vi "PupilTracker.vi"() -> ()   [LabVIEW 2013]
uses:
  PupilTrackerStates.ctl
  <vilib>/vision/NI_Vision_Development_Module.lvlib
  <vilib>/vision/Image Controls.llb/IMAQ Image.ctl
panel:
  in  "Tab Control":T1(tab)
  out "Pupil marked":bool=TRUE
  out "Saving Pupil Video":bool=TRUE
  out "LostFrames":u32
  out "Tracking Pupil":bool
  out "PupilCamera":T2(plugin-control)
  out "Frame Rate Eyetracker":dbl
  out "Avg freq":dbl caption="Eyetracker - Mean \nprocessing frequency (Hz)" format="%0.2f"
  out "Pupil Info":T3(graph)
  in  "Storage Folder":path
  in  "Save Block Video":bool
  in  "Track Pupil":bool
  in  "Rescan Image":bool=TRUE
  in  "Select Pupil Area":bool
  in  "Pupil Camera":bool=TRUE
  in  "Acquisition Frame Rate":dbl=30.0 min=1.0 max=100000.0
  out "Processed":T2(plugin-control)
  in  "Manual Threshold":cluster{sgl, sgl}(slide)={0.0, 150.0} caption="Threshold Range" scale=0.0..255.0
  in  "Track Every Nth Frame":i32=1
  in  "Exposure Time":dbl(slide)=7611.0 min=10.0 max=850000.0 scale=1000.0..10000.0
  in  "Gain":dbl(slide)=7.281634828221404 min=0.0 max=24.014274679280266 scale=0.0..10.0
  in  "Black Level":dbl(slide)=-17.75 min=-32.0 max=31.75 scale=-30.0..30.0
  in  "BtnQuit":bool
  out "Processed Image Display":T2
  out "Stop Acquisition":bool=TRUE
  out "Vision Acquisition Error":errorcluster
  out "Paused Acquisition":bool=TRUE
  out "Fitted Pupil Image":T2
  out "Last Image number":u32
  in  "Save Tracking Results":bool=TRUE
  out "Pupil Frame No":i32
  out "Processed Image":T2
  out "Cropped Image":T2
  out "Exit program":bool
  # "Camera Connection"
  # "Start Tracking"
  # "Optimize Tracking"
  # "Tracker Settings"
  # "Set tracker to rescan entire image if pupil is not found within search area"
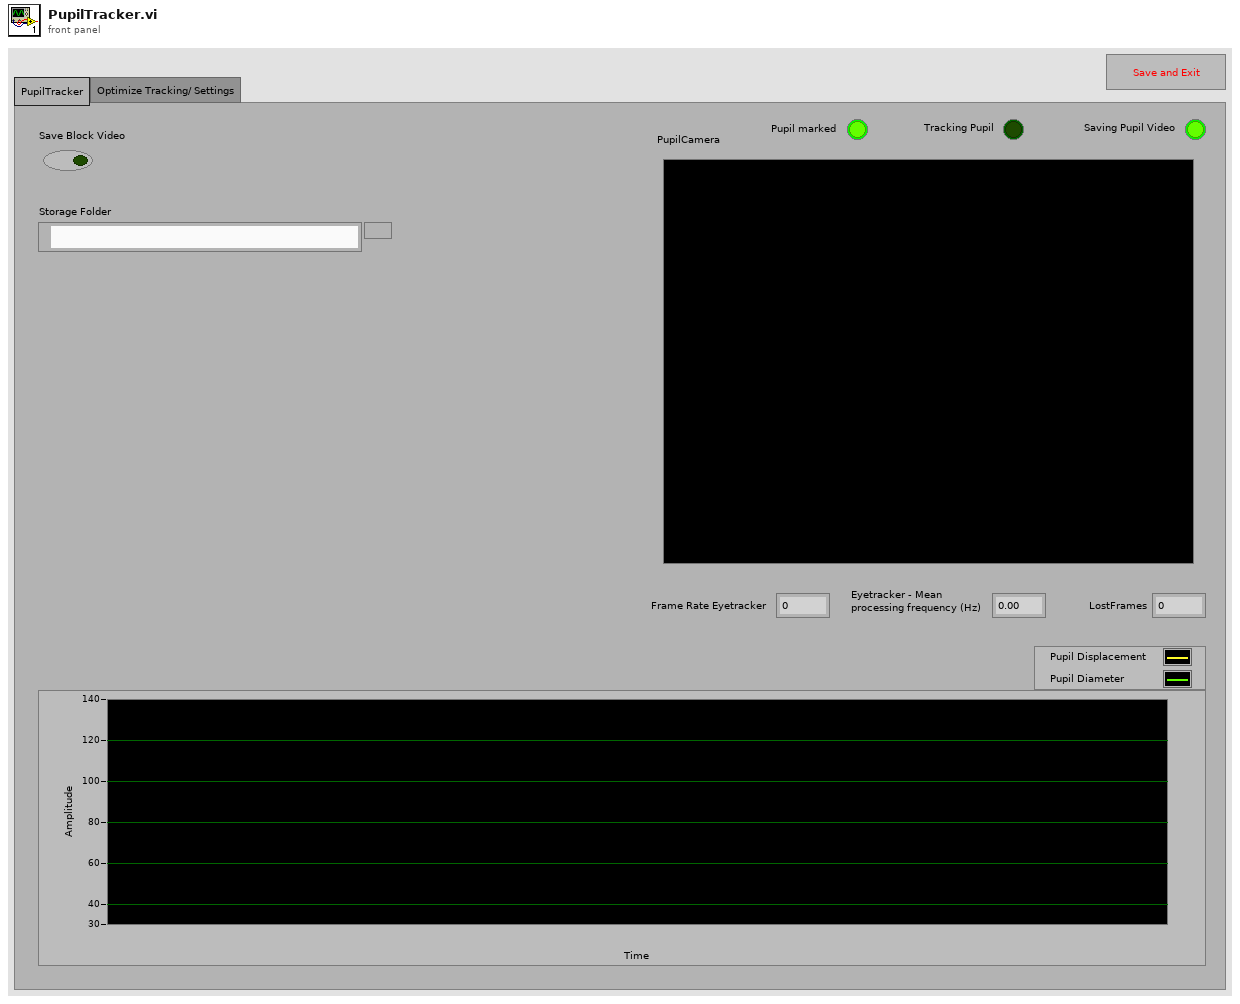
[diagram p1: front panel]
types:
  T1 = enum32{"PupilTracker", "Optimize Tracking/ Settings"}
  T2 = typedef "IMAQ Image.ctl" = refnum<image>
  T3 = cluster{"Numeric":dbl, "Average of last N array elements":dbl}
  T4 = typedef "PupilTrackerStates.ctl" = enum16{"Initialize Eyetracker", "Idle", "Run Acquisition", "Update Acquisition Parameters", "Camera Error", "Pupil Unmarked Error", "Quit Eyetracker"}
  T5 = cluster{"Numeric":dbl, "Average of last N array elements":dbl}[]
  T6 = typedef "Image Type" = u32
  T7 = cluster{"Frame No":i32, "Circle time series":dbl[][], "Rectangle coordinates":i32[], "Annulus ROI":cluster{"ID":enum32{"External", "Internal"}, "Type":u32, i32[]}, "Annulus coordinates":i32[]}
  T8 = cluster{"Pupil Displacement":dbl, "Average Pupil Diameter":dbl}
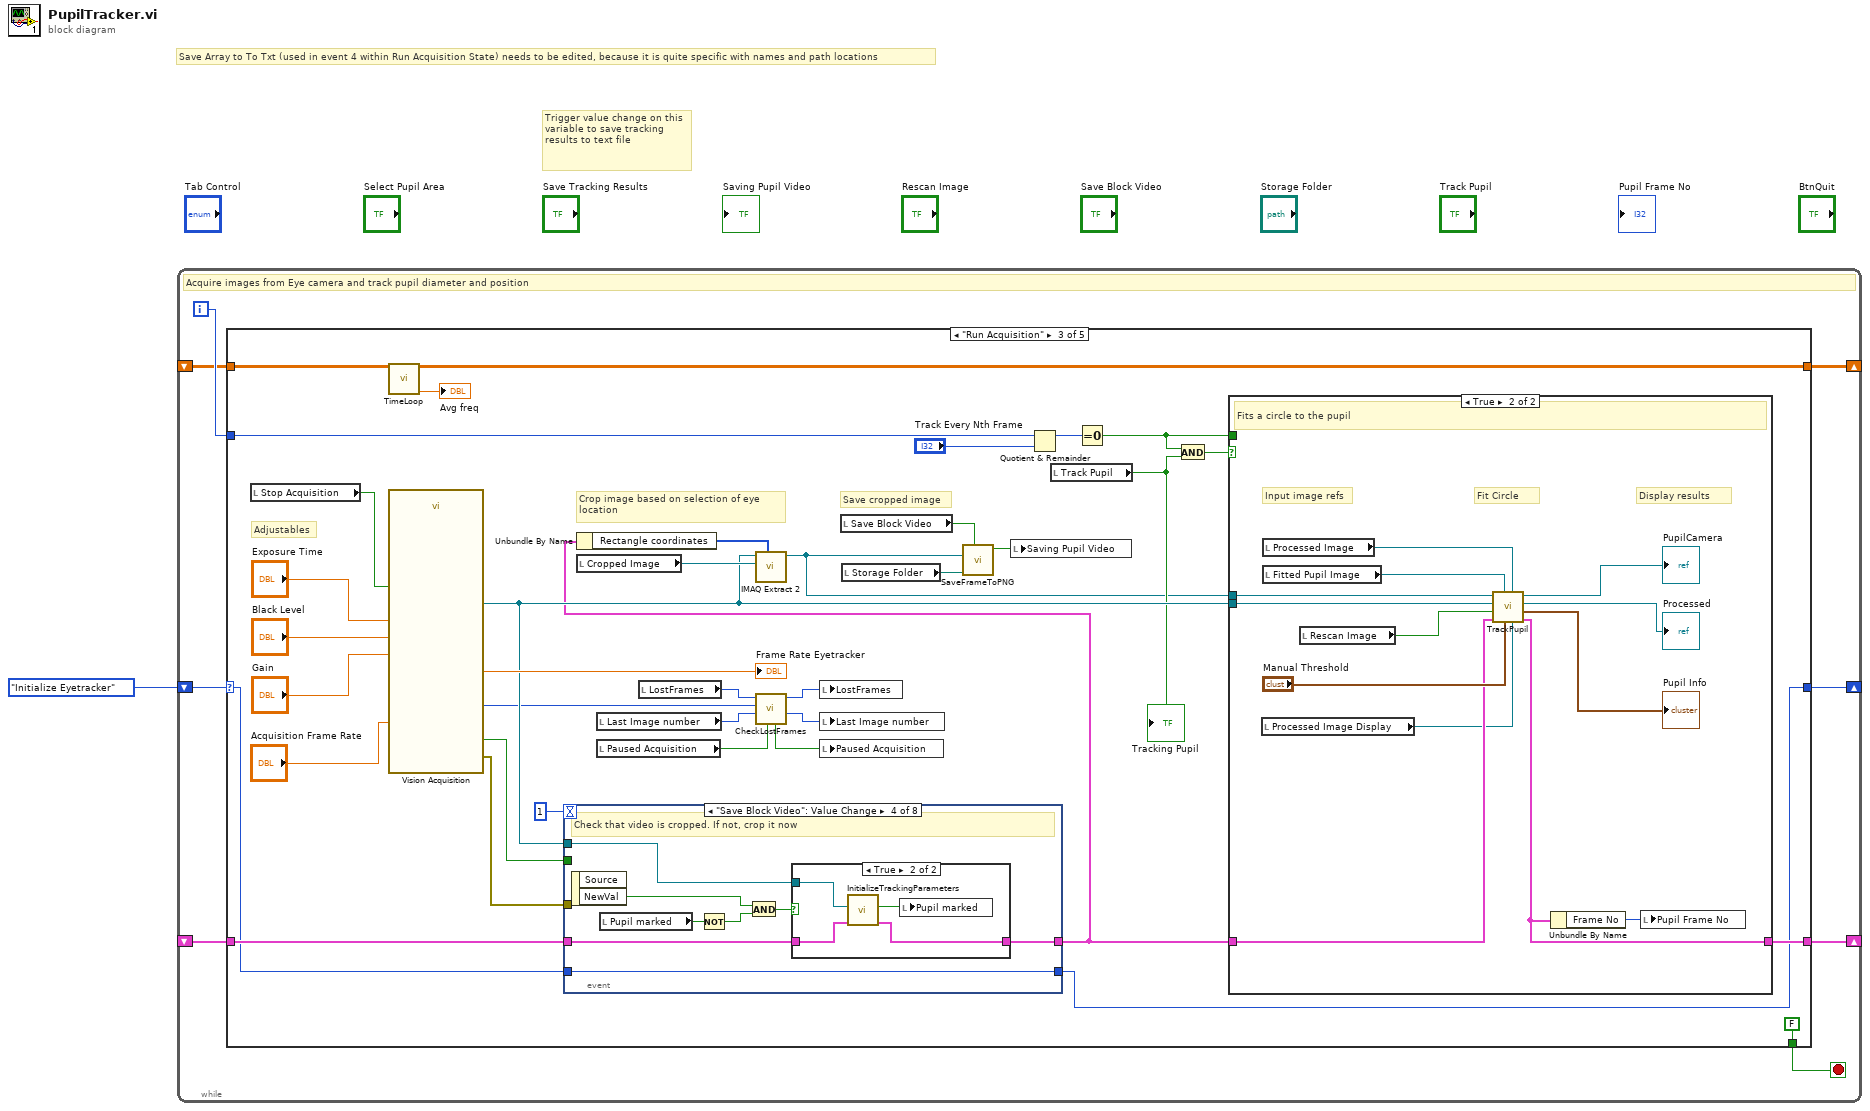
[diagram p0: block diagram]
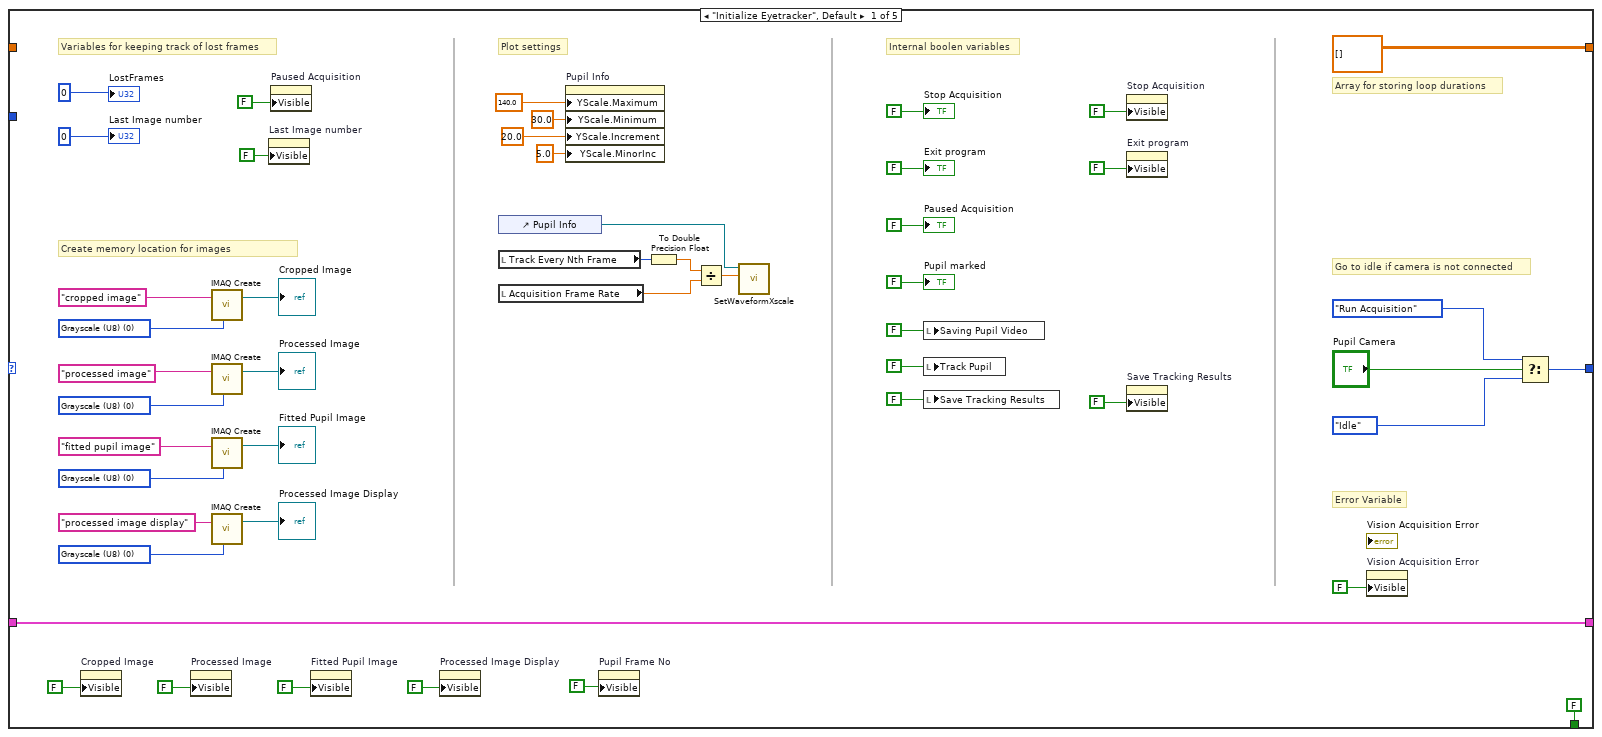
[diagram p2: hidden frame]
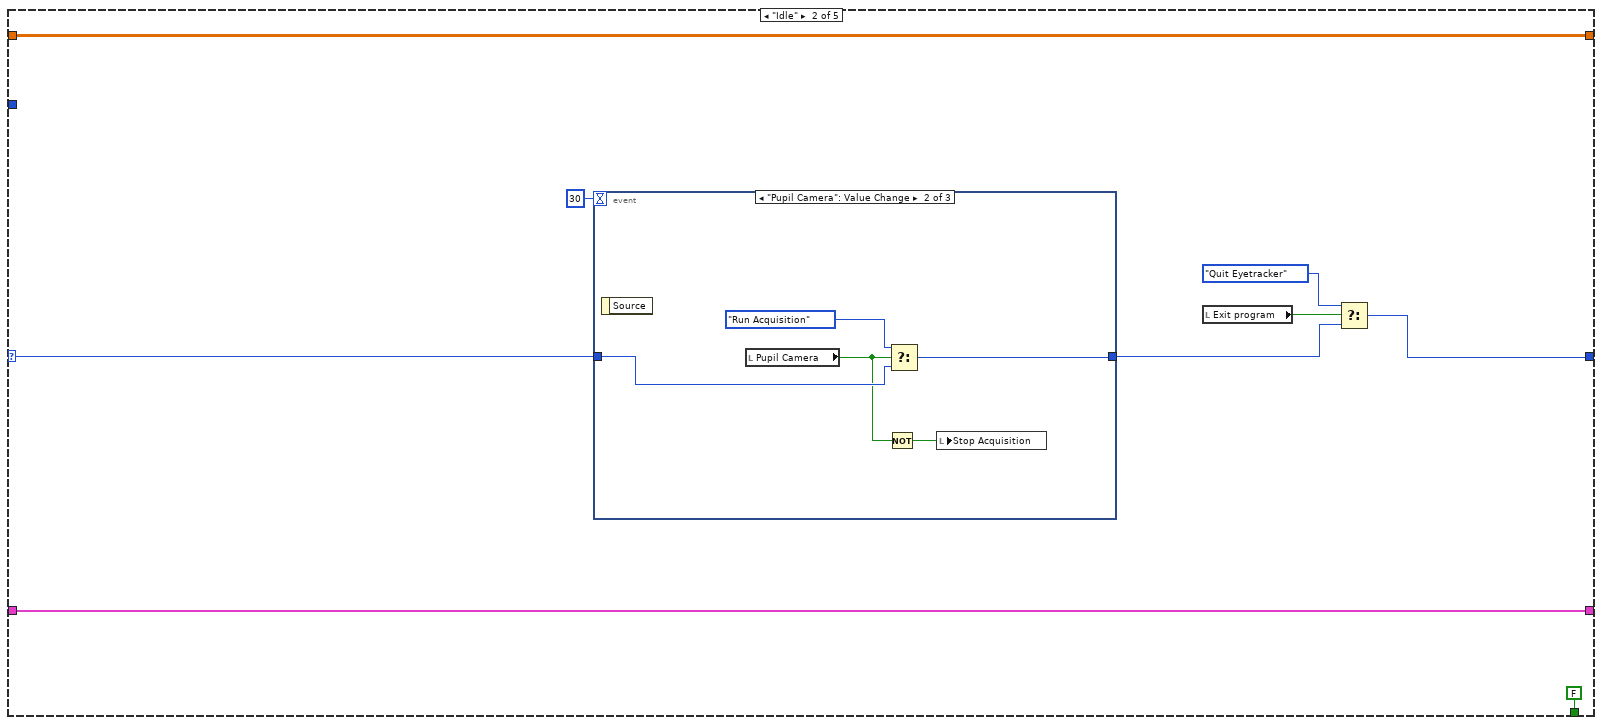
[diagram p3: hidden frame]
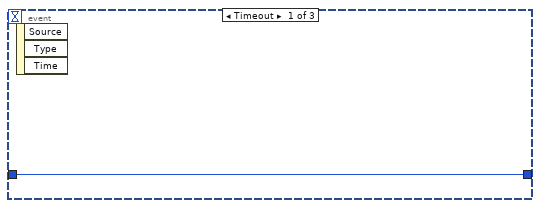
[diagram p4: hidden frame]
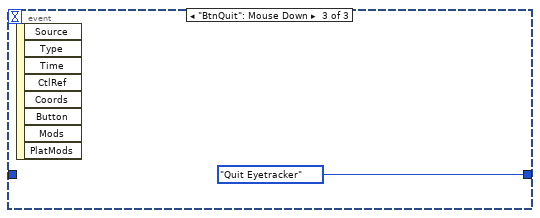
[diagram p5: hidden frame]
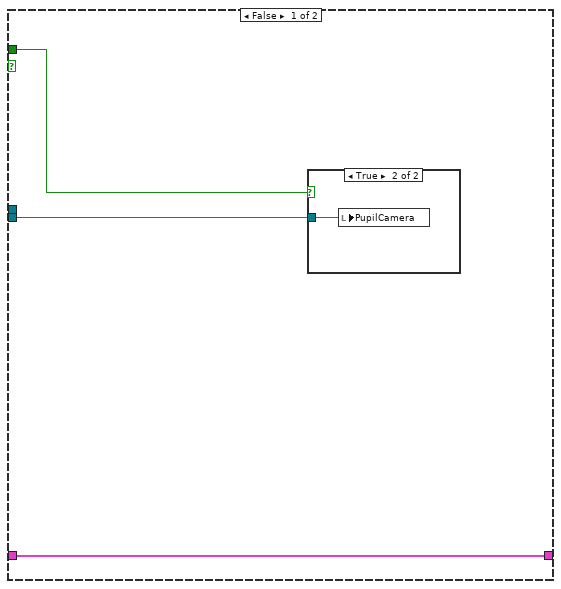
[diagram p6: hidden frame]
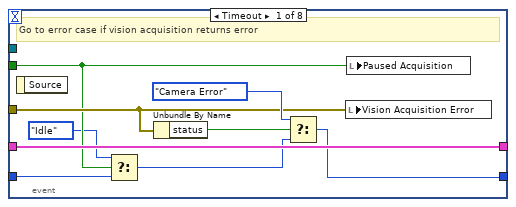
[diagram p8: hidden frame]
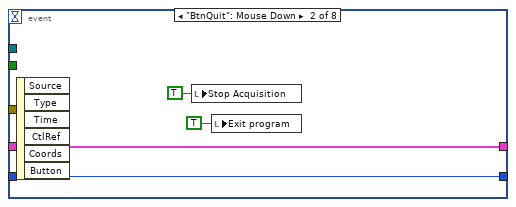
[diagram p9: hidden frame]
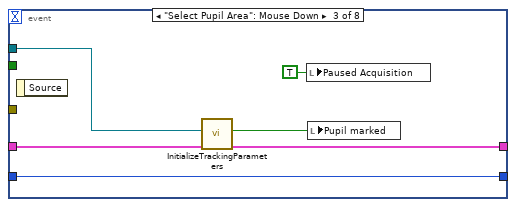
[diagram p10: hidden frame]
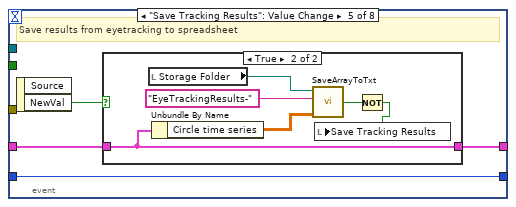
[diagram p12: hidden frame]
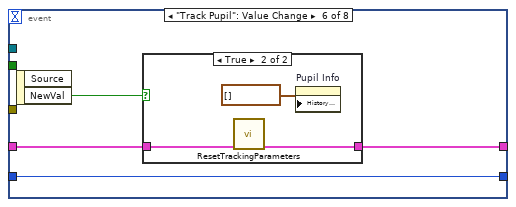
[diagram p14: hidden frame]
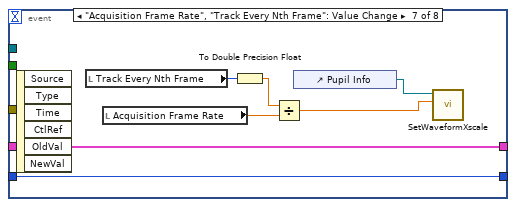
[diagram p16: hidden frame]
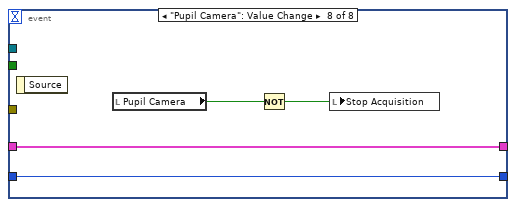
[diagram p17: hidden frame]
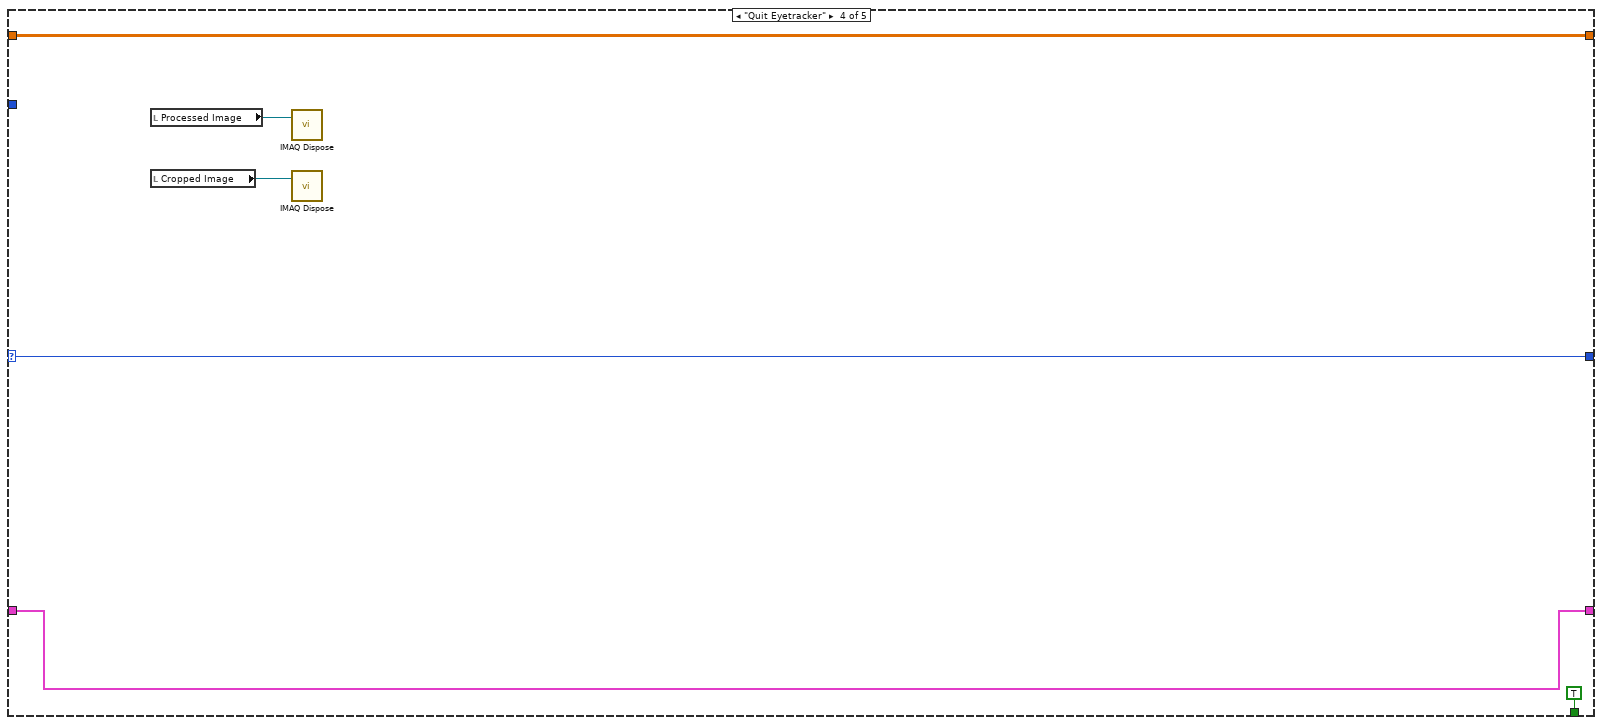
[diagram p18: hidden frame]
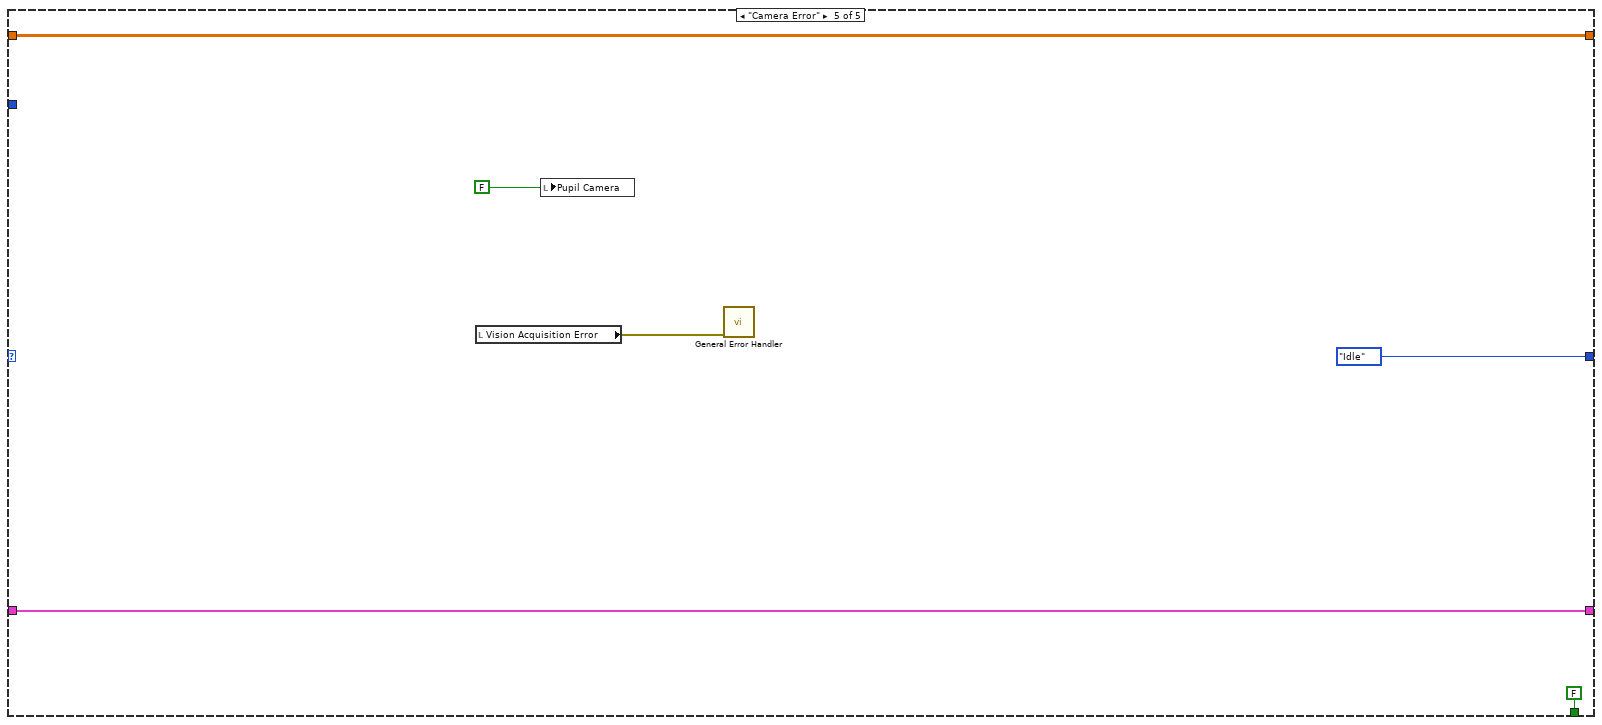
[diagram p19: hidden frame]
diagram:
  # "Save Array to To Txt (used in event 4 within Run Acquisition State) needs to be edited, because it is quite specific with names and path locations"
  # "Trigger value change on this variable to save tracking results to text file"
  n1 = while {
    shift-right: [w5] -> _
    shift-left: _ -> [w6]
    shift-right: [w9] -> _
    shift-left: _ -> [w7]
    shift-right: [w2] -> _
    shift-left: PupilTrackerStates."Initialize Eyetracker" -> [w3]
    i -> [w8]
    stop <- w4 stop-if-true
    # "Acquire images from Eye camera and track pupil diameter and position"
    n2 = case shown="\"Run Acquisition\"" w3 {
      selector: w3 -> [_ w62 w84 w193 _]
      tunnel: [w57 w65 w110 w191 w200] -> w9
      tunnel: w8 -> [_ _ w109 _ _]
      tunnel: w7 -> [w57 w65 w104 w191 w200]
      tunnel: w6 -> [_ w66 w92 w196 w201]
      tunnel: [dbl[][] [] w66 w91 w196 w201] -> w5
      tunnel: [w55 w59 w83 w193 PupilTrackerStates."Idle"] -> w2
      tunnel: [FALSE ("Stopped") FALSE ("Stopped") FALSE ("Stopped") TRUE ("Stopped") FALSE ("Stopped")] -> w4
      frame "Initialize Eyetracker", Default {
        w29 = T6 0 items=["Grayscale (U8)", "Grayscale (I16)", "Grayscale (SGL)", "Complex (CSG)", "RGB (U32)", "HSL (U32)", "RGB (U64)", "Grayscale (U16)"] ("Image Type")
        w48 = T6 0 items=["Grayscale (U8)", "Grayscale (I16)", "Grayscale (SGL)", "Complex (CSG)", "RGB (U32)", "HSL (U32)", "RGB (U64)", "Grayscale (U16)"] ("Image Type")
        w51 = T6 0 items=["Grayscale (U8)", "Grayscale (I16)", "Grayscale (SGL)", "Complex (CSG)", "RGB (U32)", "HSL (U32)", "RGB (U64)", "Grayscale (U16)"] ("Image Type")
        w53 = T6 0 items=["Grayscale (U8)", "Grayscale (I16)", "Grayscale (SGL)", "Complex (CSG)", "RGB (U32)", "HSL (U32)", "RGB (U64)", "Grayscale (U16)"] ("Image Type")
        # "Error Variable"
        # "Internal boolen variables"
        # "Plot settings"
        # "Go to idle if camera is not connected"
        # "Variables for keeping track of lost frames"
        # "Create memory location for images"
        # "Array for storing loop durations"
        n3 = property on="Cropped Image" class="IMAQImage (strict)"("Visible"=FALSE) -> ()  [unwired: 2 in, 2 out]
        n4 = property on="Processed Image" class="IMAQImage (strict)"("Visible"=FALSE) -> ()  [unwired: 2 in, 2 out]
        n5 = call "IMAQ Create"("Image Name"="cropped image", "Image Type"=w53) -> ("New Image"=→"Cropped Image":T2)  [unwired: 3 in, 1 out]
        n6 = call "IMAQ Create"("Image Name"="processed image", "Image Type"=w51) -> ("New Image"=→"Processed Image":T2)  [unwired: 3 in, 1 out]
        n7 = call "IMAQ Create"("Image Name"="fitted pupil image", "Image Type"=w48) -> ("New Image"=→"Fitted Pupil Image":T2)  [unwired: 3 in, 1 out]
        n8 = call "IMAQ Create"("Image Name"="processed image display", "Image Type"=w29) -> ("New Image"=→"Processed Image Display":T2)  [unwired: 3 in, 1 out]
        n9 = property on="Last Image number" class="DigNum (strict)"("Visible"=FALSE) -> ()  [unwired: 2 in, 2 out]
        n10 = property on="Paused Acquisition" class="Bool (strict)"("Visible"=FALSE) -> ()  [unwired: 2 in, 2 out]
        n11 = property on="Fitted Pupil Image" class="IMAQImage (strict)"("Visible"=FALSE) -> ()  [unwired: 2 in, 2 out]
        n12 = property on="Processed Image Display" class="IMAQImage (strict)"("Visible"=FALSE) -> ()  [unwired: 2 in, 2 out]
        n13 = control-ref of="Pupil Info"() -> (w30:refnum<vi>)
        n14 = local read "Track Every Nth Frame"() -> (w40:i32)
        n15 = local read "Acquisition Frame Rate"() -> (w41:dbl)
        n16 = property on="Pupil Info" class="WFChart (strict)"("YScale.Maximum"=140.0 ("Y Scale.Range:Increment"), "YScale.Minimum"=30.0 ("Y Scale.Range:Maximum"), "YScale.Increment"=20.0 ("Y Scale.Range:Minimum"), "YScale.MinorInc"=5.0 ("Y Scale.Range:Minor Increment")) -> ()  [unwired: 2 in, 2 out]
        n17 = property on="Pupil Frame No" class="DigNum (strict)"("Visible"=FALSE) -> ()  [unwired: 2 in, 2 out]
        n18 = To Double Precision Float(number=w40) -> (double precision float=w39:dbl)
        n19 = Divide(x=w39, y=w41) -> (x/y=w33:dbl)
        n20 = call "SetWaveformXscale.vi"("deltaT"=w33, "WaveformChart in"=w30) -> ()  [unwired: 10 in]
        n21 = local write "Saving Pupil Video"(FALSE ("Saving Pupil Video")) -> ()
        n22 = local write "Track Pupil"(FALSE ("Track Pupil")) -> ()
        n23 = local write "Save Tracking Results"(FALSE ("Save Tracking Results")) -> ()
        n24 = property on="Stop Acquisition" class="Bool (strict)"("Visible"=FALSE) -> ()  [unwired: 2 in, 2 out]
        n25 = property on="Exit program" class="Bool (strict)"("Visible"=FALSE) -> ()  [unwired: 2 in, 2 out]
        n26 = property on="Save Tracking Results" class="Bool (strict)"("Visible"=FALSE) -> ()  [unwired: 2 in, 2 out]
        n27 = property on="Vision Acquisition Error" class="Clust (strict)"("Visible"=FALSE) -> ()  [unwired: 2 in, 2 out]
        n28 = Select(t=PupilTrackerStates."Run Acquisition", s="Pupil Camera", f=PupilTrackerStates."Idle") -> (s? t:f=w55:T4)
        "Last Image number" <- u32 0 ("Last Image number")
        "LostFrames" <- u32 0 ("LostFrames")
        "Paused Acquisition" <- FALSE ("Paused Acquisition")
        "Exit program" <- FALSE ("Exit program")
        "Stop Acquisition" <- FALSE ("Stop Acquisition")
        "Pupil marked" <- FALSE ("Pupil marked")
      }
      frame "Idle" {
        n29 = event shown="[1] \"Pupil Camera\": Value Change" {
          selector: _ -> [_ _ _]
          dyn-events: _ -> [_ _ _]
          timeout: 30 -> [_ _ _]
          tunnel: [w67 w72 PupilTrackerStates."Quit Eyetracker"] -> w60
          tunnel: w62 -> [w67 w71 _]
          event Timeout {
            n30 = event-data() -> ()  [unwired: 1 in, 3 out]
          }
          event "Pupil Camera": Value Change {
            n31 = event-data() -> ()  [unwired: 1 in, 1 out]
            n32 = local read "Pupil Camera"() -> (w68:bool)
            n33 = Not(x=w68) -> (.not. x?=w69:bool)
            n34 = Select(t=PupilTrackerStates."Run Acquisition", s=w68, f=w71) -> (s? t:f=w72:T4)
            n35 = local write "Stop Acquisition"(w69) -> ()
          }
          event "BtnQuit": Mouse Down {
            n36 = event-data() -> ()  [unwired: 1 in, 8 out]
          }
        }
        n37 = local read "Exit program"() -> (w61:bool)
        n38 = Select(t=PupilTrackerStates."Quit Eyetracker", s=w61, f=w60) -> (s? t:f=w59:T4)
      }
      frame "Run Acquisition" {
        # "Save cropped image"
        # "Crop image based on selection of eye location"
        # "Adjustables"
        n39 = local read "Stop Acquisition"() -> (w79:bool)
        n40 = call "TimeLoop.vi"("Loop durations in"=w92) -> ("Average fps"=→"Avg freq":dbl, "Loop durations out"=w91:dbl[][])  [unwired: 5 in]
        n41 = call "Vision Acquisition"("Analog Control::Gain"="Gain", "Analog Control::Black Level"="Black Level", "Acquisition Control::Exposure Time"="Exposure Time", "Acquisition Control::Acquisition Frame Rate"="Acquisition Frame Rate", "Stop (F)"=w79) -> ("Image Out"=w100:T2, "Image Number"=w96:u32, "Frame Rate"=→"Frame Rate Eyetracker":dbl, "Stopped"=w82:bool, "error out"=w78:errorcluster)  [unwired: 17 in, 1 out]
        n42 = event shown="[3] \"Save Block Video\": Value Change" {
          selector: _ -> [_ _ _ _ _ _ _ _]
          dyn-events: _ -> [_ _ _ _ _ _ _ _]
          timeout: 1 -> [_ _ _ _ _ _ _ _]
          tunnel: w100 -> [_ _ w147 w155 _ _ _ _]
          tunnel: w104 -> [w137 w141 w146 w154 w164 w174 w185 w190]
          tunnel: [w137 w141 w145 w153 w163 w173 w185 w190] -> w90
          tunnel: w84 -> [w130 w140 w143 w148 w161 w172 w186 w189]
          tunnel: [w131 w140 w143 w148 w161 w172 w186 w189] -> w83
          tunnel: w82 -> [w133 _ _ _ _ _ _ _]
          tunnel: w78 -> [w134 _ _ _ _ _ _ _]
          event Timeout {
            # "Go to error case if vision acquisition returns error"
            n43 = event-data() -> ()  [unwired: 1 in, 1 out]
            n44 = Select(t=PupilTrackerStates."Idle", s=w133, f=w130) -> (s? t:f=w129:T4)
            n45 = Unbundle By Name(w134) -> ("status"=w136:bool)
            n46 = Select(t=PupilTrackerStates."Camera Error", s=w136, f=w129) -> (s? t:f=w131:T4)
            n47 = local write "Vision Acquisition Error"(w134) -> ()
            n48 = local write "Paused Acquisition"(w133) -> ()
          }
          event "BtnQuit": Mouse Down {
            n49 = event-data() -> ()  [unwired: 1 in, 6 out]
            n50 = local write "Stop Acquisition"(TRUE ("Stop Acquisition")) -> ()
            n51 = local write "Exit program"(TRUE ("Exit program")) -> ()
          }
          event "Select Pupil Area": Mouse Down {
            n52 = event-data() -> ()  [unwired: 1 in, 1 out]
            n53 = call "InitializeTrackingParameters.vi"("Circle fit parameters in"=w146, "Refnum in"=w147) -> ("Circle fit parameters out"=w145:T7, "Pupil Marked"=w144:bool)  [unwired: 4 in]
            n54 = local write "Paused Acquisition"(TRUE ("Paused Acquisition")) -> ()
            n55 = local write "Pupil marked"(w144) -> ()
          }
          event "Save Block Video": Value Change {
            # "Check that video is cropped. If not, crop it now"
            n56 = event-data() -> ("NewVal"=w149:bool)  [unwired: 1 in, 1 out]
            n57 = local read "Pupil marked"() -> (w151:bool)
            n58 = Not(x=w151) -> (.not. x?=w152:bool)
            n59 = And(x=w149, y=w152) -> (x .and. y?=w150:bool)
            n60 = case shown="True" w150 {
              tunnel: w155 -> [_ w159]
              tunnel: w154 -> [w156 w158]
              tunnel: [w156 w157] -> w153
              frame False {
              }
              frame True {
                n61 = call "InitializeTrackingParameters.vi"("Circle fit parameters in"=w158, "Refnum in"=w159) -> ("Circle fit parameters out"=w157:T7, "Pupil Marked"=w160:bool)  [unwired: 4 in]
                n62 = local write "Pupil marked"(w160) -> ()
              }
            }
          }
          event "Save Tracking Results": Value Change {
            # "Save results from eyetracking to spreadsheet"
            n63 = event-data() -> ("NewVal"=w162:bool)  [unwired: 1 in, 1 out]
            n64 = case shown="True" w162 {
              tunnel: w164 -> [w165 w168]
              tunnel: [w165 w168] -> w163
              frame False {
              }
              frame True {
                n65 = local read "Storage Folder"() -> (w171:path)
                n66 = Unbundle By Name(w168) -> ("Circle time series"=w169:dbl[][])
                n67 = call "SaveArrayToTxt.vi"("Input array"=w169, "Filename"="EyeTrackingResults-", "File path"=w171) -> ("Boolean"=w167:bool)  [unwired: 1 in]
                n68 = Not(x=w167) -> (.not. x?=w166:bool)
                n69 = local write "Save Tracking Results"(w166) -> ()
              }
            }
          }
          event "Track Pupil": Value Change {
            n70 = event-data() -> ("NewVal"=w175:bool)  [unwired: 1 in, 1 out]
            n71 = case shown="True" w175 {
              tunnel: w174 -> [w176 w179]
              tunnel: [w176 w178] -> w173
              frame False {
              }
              frame True {
                n72 = call "ResetTrackingParameters.vi"("tracking parameters in"=w179) -> ("tracking parameters out"=w178:T7)  [unwired: 10 in]
                n73 = property on="Pupil Info" class="WFChart (strict)"("History Data"=T5 []) -> ()  [unwired: 2 in, 2 out]
              }
            }
          }
          event "Acquisition Frame Rate", "Track Every Nth Frame": Value Change {
            n74 = event-data() -> ()  [unwired: 1 in, 6 out]
            n75 = local read "Track Every Nth Frame"() -> (w183:i32)
            n76 = local read "Acquisition Frame Rate"() -> (w184:dbl)
            n77 = To Double Precision Float(number=w183) -> (double precision float=w182:dbl)
            n78 = Divide(x=w182, y=w184) -> (x/y=w181:dbl)
            n79 = control-ref of="Pupil Info"() -> (w180:refnum<vi>)
            n80 = call "SetWaveformXscale.vi"("deltaT"=w181, "WaveformChart in"=w180) -> ()  [unwired: 10 in]
          }
          event "Pupil Camera": Value Change {
            n81 = event-data() -> ()  [unwired: 1 in, 1 out]
            n82 = local read "Pupil Camera"() -> (w188:bool)
            n83 = Not(x=w188) -> (.not. x?=w187:bool)
            n84 = local write "Stop Acquisition"(w187) -> ()
          }
        }
        n85 = Unbundle By Name(w90) -> ("Rectangle coordinates"=w106:i32[])
        n86 = local read "Cropped Image"() -> (w107:T2)
        n87 = local read "Last Image number"() -> (w93:u32)
        n88 = local read "Paused Acquisition"() -> (w88:bool)
        n89 = local read "LostFrames"() -> (w94:u32)
        n90 = call "IMAQ Extract 2"("Optional Rectangle"=w106, "Image Dst"=w107, "Image Src"=w100) -> ("Image Dst Out"=w77:T2)  [unwired: 7 in, 1 out]
        n91 = call "CheckLostFrames.vi"("Pause Acquisition in"=w88, "Last Image number"=w93, "Image Number"=w96, "LostFrames in"=w94) -> ("Last Image Number"=w89:u32, "LostFrames out"=w95:u32, "Pause Acquisition out"=w87:bool)  [unwired: 5 in]
        n92 = local write "LostFrames"(w95) -> ()
        n93 = local write "Last Image number"(w89) -> ()
        n94 = local write "Paused Acquisition"(w87) -> ()
        n95 = local read "Save Block Video"() -> (w76:bool)
        n96 = local read "Storage Folder"() -> (w74:path)
        n97 = call "SaveFrameToPNG.vi"("Save Image?"=w76, "Block Folder"=w74, "Refnum in"=w77) -> ("ImageSaved"=w75:bool)  [unwired: 7 in, 1 out]
        n98 = local write "Saving Pupil Video"(w75) -> ()
        n99 = Quotient & Remainder(x=w109, y="Track Every Nth Frame") -> (x-y*floor(x/y)=w105:i32)  [unwired: 1 out]
        n100 = local read "Track Pupil"() -> (w85:bool)
        "Tracking Pupil" <- w85
        n101 = Equal To 0?(x=w105) -> (x = 0?=w86:bool)
        n102 = And(x=w86, y=w85) -> (x .and. y?=w102:bool)
        n103 = case shown="True" w102 {
          tunnel: w100 -> [w114 w121]
          tunnel: w90 -> [w113 w124]
          tunnel: [w113 w123] -> w110
          tunnel: w77 -> [_ w122]
          tunnel: w86 -> [w112 _]
          frame False {
            n104 = case shown="True" w112 {
              tunnel: w114 -> [_ w115]
              frame False {
              }
              frame True {
                n105 = local write "PupilCamera"(w115) -> ()
              }
            }
          }
          frame True {
            # "Input image refs"
            # "Display results"
            # "Fit Circle"
            # "Fits a circle to the pupil"
            n106 = local read "Processed Image Display"() -> (w117:T2)
            n107 = local read "Processed Image"() -> (w126:T2)
            n108 = local read "Fitted Pupil Image"() -> (w119:T2)
            n109 = local read "Rescan Image"() -> (w120:bool)
            n110 = call "TrackPupil.vi"("Processed image display refnum"=w117, "Processed image"=w126, "Manual Threshold"="Manual Threshold", "Fitted image refnum"=w119, "Circle fit parameters in"=w124, "Rescan image if pupil is lost"=w120, "Acquired image refnum"=w121, "Cropped image refnum"=w122) -> ("Circle fit parameters out"=w123:T7, "New Values"=→"Pupil Info":T8, "Processed image display refnum out"=→"Processed":T2, "Fitted image refnum out"=→"PupilCamera":T2)
            n111 = Unbundle By Name(w123) -> ("Frame No"=w127:i32)
            n112 = local write "Pupil Frame No"(w127) -> ()
          }
        }
      }
      frame "Quit Eyetracker" {
        n113 = local read "Processed Image"() -> (w195:T2)
        n114 = local read "Cropped Image"() -> (w194:T2)
        n115 = call "IMAQ Dispose"("Image"=w195) -> ()  [unwired: 5 in, 1 out]
        n116 = call "IMAQ Dispose"("Image"=w194) -> ()  [unwired: 5 in, 1 out]
      }
      frame "Camera Error" {
        n117 = local read "Vision Acquisition Error"() -> (w197:errorcluster)
        n118 = local write "Pupil Camera"(FALSE ("Eye Tracking Camera")) -> ()
        n119 = call <vilib>:"General Error Handler.vi"("error in (no error)"=w197) -> ()  [unwired: 10 in, 5 out]
      }
    }
  }
